vi "Index Boolean Tag.vi"(4 "Write?":bool, 6 "Default Value":bool, 8 "error in (no error)":errorcluster, 9 "Tag":string, 10 "Group Index":i32, 11 "bt_Blackboard in":refnum<class "bt_Blackboard.lvclass">) -> (0 "error out":errorcluster, 1 "New Tag?":bool, 2 "Index":i32, 3 "bt_Blackboard out":refnum<class "bt_Blackboard.lvclass">)   [LabVIEW 2021, in "BT.lvlib" / "bt_Blackboard.lvclass"]
uses:
  bt_Blackboard.lvclass
  bt_Blackboard.lvclass/bt_Blackboard.ctl
  Status Type.ctl
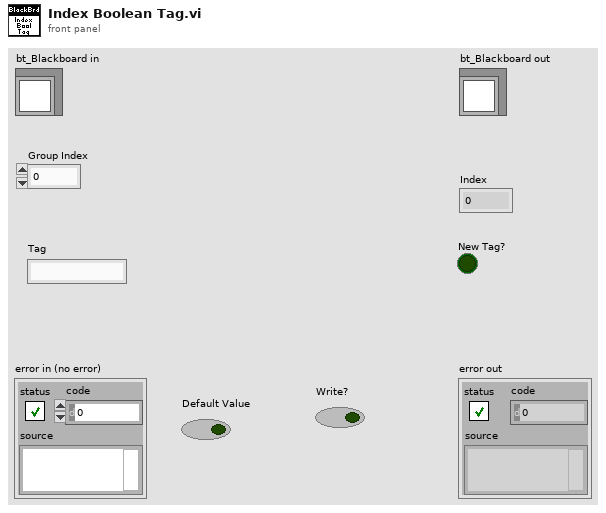
[diagram p1: front panel]
types:
  T1 = typedef "BT.lvlib/bt_Blackboard.lvclass/Status Type.ctl" = cluster{"Read?":bool, "Write?":bool}
  T2 = typedef "BT.lvlib/bt_Blackboard.lvclass/Data DVR Type.ctl" = cluster{"Boolean":cluster{"Tags":refnum<data-value>, "Boolean":refnum<data-value>, "Status":refnum<data-value>}, "String":cluster{"Tags":refnum<data-value>, "String":refnum<data-value>, "Status":refnum<data-value>}, "DBL":cluster{"Tags":refnum<data-value>, "DBL":refnum<data-value>, "Status":refnum<data-value>}, "SGL":cluster{"Tags":refnum<data-value>, "SGL":refnum<data-value>, "Status":refnum<data-value>}, "EXT":cluster{"Tags":refnum<data-value>, "EXT":refnum<data-value>, "Status":refnum<data-value>}, "U8":cluster{"Tags":refnum<data-value>, "U8":refnum<data-value>, "Status":refnum<data-value>}, "U16":cluster{"Tags":refnum<data-value>, "U16":refnum<data-value>, "Status":refnum<data-value>}, "U32":cluster{"Tags":refnum<data-value>, "U32":refnum<data-value>, "Status":refnum<data-value>}, "U64":cluster{"Tags":refnum<data-value>, "U64":refnum<data-value>, "Status":refnum<data-value>}, "I8":cluster{"Tags":refnum<data-value>, "I8":refnum<data-value>, "Status":refnum<data-value>}, "I16":cluster{"Tags":refnum<data-value>, "I16":refnum<data-value>, "Status":refnum<data-value>}, "I32":cluster{"Tags":refnum<data-value>, "I32":refnum<data-value>, "Status":refnum<data-value>}, "I64":cluster{"Tags":refnum<data-value>, "I64":refnum<data-value>, "Status":refnum<data-value>}, "CDBL":cluster{"Tags":refnum<data-value>, "CDBL":refnum<data-value>, "Status":refnum<data-value>}, "CSGL":cluster{"Tags":refnum<data-value>, "CSGL":refnum<data-value>, "Status":refnum<data-value>}, "CEXT":cluster{"Tags":refnum<data-value>, "CEXT":refnum<data-value>, "Status":refnum<data-value>}, "Time":cluster{"Tags":refnum<data-value>, "Time":refnum<data-value>}, "Variant":cluster{"Tags":refnum<data-value>, "Variant":refnum<data-value>, "Status":refnum<data-value>}, "Waveform":cluster{"Tags":refnum<data-value>, "Waveform":refnum<data-value>, "Status":refnum<data-value>}}
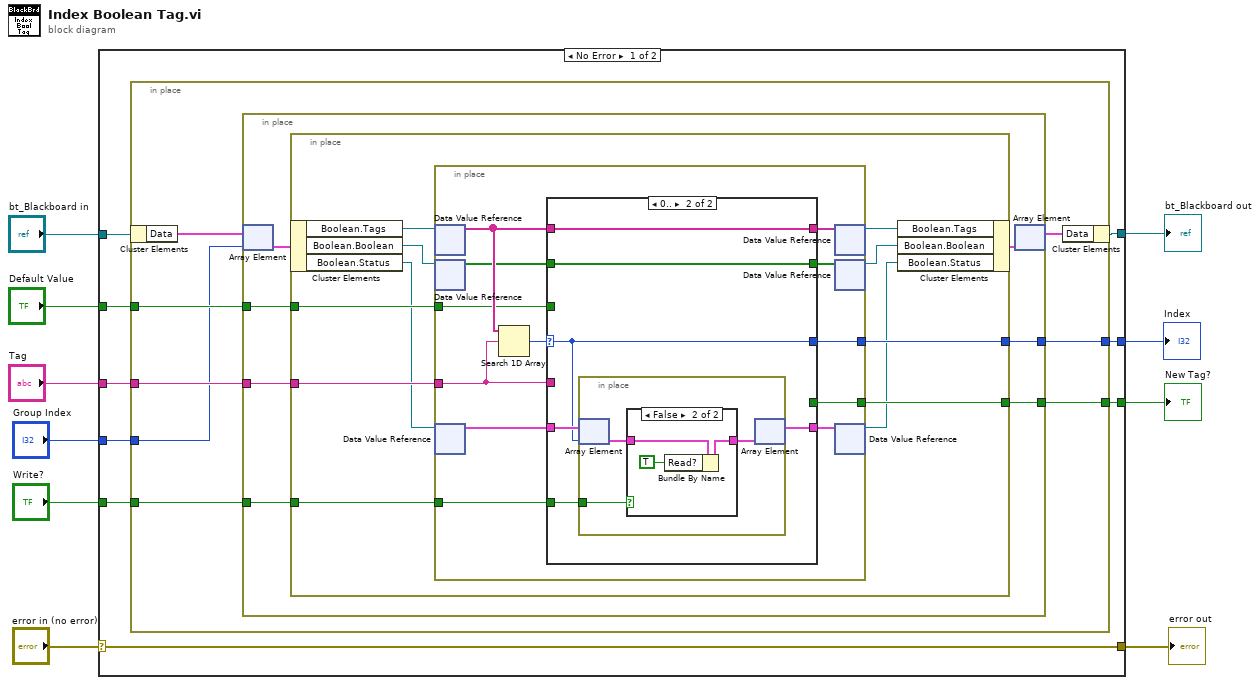
[diagram p0: block diagram]
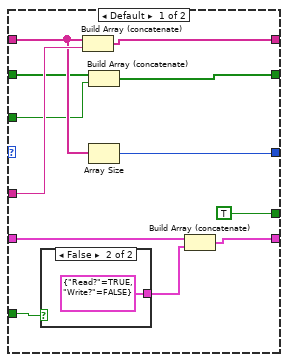
[diagram p2: hidden frame]
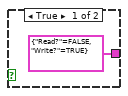
[diagram p3: hidden frame]
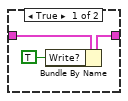
[diagram p4: hidden frame]
diagram:
  n1 = case shown="No Error" "error in (no error)" {
    selector: "error in (no error)" -> [w18 w88]
    tunnel: [w18 w88] -> w9
    tunnel: [w13 w87] -> w7
    tunnel: "bt_Blackboard in" -> [w14 w87]
    tunnel: "Tag" -> [w19 _]
    tunnel: [w17 _] -> w5
    tunnel: [w16 _] -> w4
    tunnel: "Default Value" -> [w15 _]
    tunnel: "Group Index" -> [w12 _]
    tunnel: "Write?" -> [w11 _]
    frame No Error {
      n2 = in-place {
        in-place-border: w19 -> [w27]
        in-place-border: [w26] -> w17
        in-place-border: [w25] -> w16
        in-place-border: w15 -> [w24]
        in-place-border: w12 -> [w21]
        in-place-border: w11 -> [w20]
        n3 = in-place-cluster #1(w14) -> ("Data"=w23:T2[])
        n4 = in-place {
          in-place-border: w27 -> [w34]
          in-place-border: [w33] -> w26
          in-place-border: [w32] -> w25
          in-place-border: w24 -> [w31]
          in-place-border: w20 -> [w28]
          n5 = in-place-array #2(w23, w21) -> (w30:T2)
          n6 = in-place {
            in-place-border: w34 -> [w43]
            in-place-border: [w42] -> w33
            in-place-border: [w41] -> w32
            in-place-border: w31 -> [w40]
            in-place-border: w28 -> [w36]
            n7 = in-place-cluster #3(w30) -> ("Boolean.Tags"=w45:refnum<data-value>, "Boolean.Boolean"=w39:refnum<data-value>, "Boolean.Status"=w37:refnum<data-value>)
            n8 = in-place {
              in-place-border: w43 -> [w54]
              in-place-border: [w53] -> w42
              in-place-border: [w52] -> w41
              in-place-border: w40 -> [w51]
              in-place-border: w36 -> [w46]
              n9 = in-place-dvr #4(w45) -> (w56:string[])  [unwired: 1 out]
              n10 = in-place-dvr #5(w39) -> (w50:bool[])  [unwired: 1 out]
              n11 = in-place-dvr #6(w37) -> (w48:T1[])  [unwired: 1 out]
              n12 = Search 1D Array(1D array=w56, element=w54) -> (index of element=w57:i32)  [unwired: 1 in]
              n13 = case shown="0.." w57 {
                selector: w57 -> [_ w73]
                tunnel: w56 -> [w67 w77]
                tunnel: [w69 w77] -> w55
                tunnel: w54 -> [w68 _]
                tunnel: [w66 w73] -> w53
                tunnel: [TRUE _] -> w52
                tunnel: w50 -> [w63 w76]
                tunnel: w51 -> [w64 _]
                tunnel: [w62 w76] -> w49
                tunnel: w48 -> [w61 w75]
                tunnel: [w60 w74] -> w47
                tunnel: w46 -> [w58 w72]
                frame Default {
                  n14 = case shown="False" w58 {
                    tunnel: [T1 {"Read?"=FALSE, "Write?"=TRUE} ("Status") T1 {"Read?"=TRUE, "Write?"=FALSE} ("Status")] -> w59
                    frame True {
                    }
                    frame False {
                    }
                  }
                  n15 = Build Array (concatenate)(w67, w68) -> (w69:string[])
                  n16 = Build Array (concatenate)(w63, w64) -> (w62:bool[])
                  n17 = Array Size(array=w67) -> (size(s)=w66:i32)
                  n18 = Build Array (concatenate)(w61, w59) -> (w60:T1[])
                }
                frame 0.. {
                  n19 = in-place {
                    in-place-border: w72 -> [w80]
                    n20 = in-place-array #7(w75, w73) -> (w79:T1)
                    n21 = case shown="False" w80 {
                      tunnel: w79 -> [w83 w86]
                      tunnel: [w82 w85] -> w78
                      frame True {
                        n22 = Bundle By Name(cluster=w83, "Write?"=TRUE) -> (w82:T1)
                      }
                      frame False {
                        n23 = Bundle By Name(cluster=w86, "Read?"=TRUE ("Write?")) -> (w85:T1)
                      }
                    }
                    n24 = in-place-array #7(w78) -> (w74:T1[])  [unwired: 1 out]
                  }
                }
              }
              n25 = in-place-dvr #4(w55) -> (w44:refnum<data-value>)  [unwired: 1 out]
              n26 = in-place-dvr #5(w49) -> (w38:refnum<data-value>)  [unwired: 1 out]
              n27 = in-place-dvr #6(w47) -> (w35:refnum<data-value>)  [unwired: 1 out]
            }
            n28 = in-place-cluster #3("Boolean.Tags"=w44, "Boolean.Boolean"=w38, "Boolean.Status"=w35) -> (w29:T2)
          }
          n29 = in-place-array #2(w29) -> (w22:T2[])  [unwired: 1 out]
        }
        n30 = in-place-cluster #1("Data"=w22) -> (w13:refnum<class "bt_Blackboard.lvclass">)
      }
    }
    frame Error {
    }
  }
  "error out" <- w9
  "bt_Blackboard out" <- w7
  "Index" <- w5
  "New Tag?" <- w4
